vi "LS218_AIDE.vi"() -> ()   [LabVIEW 2014]
panel:
  in  "Bouton OK":bool
  # "VÉRIFICATION DU DÉBIT DU LAKESHORE 218:"
  # "Le débit doit être le même entre le LS218 et le logiciel d'acquisition"
  # "VÉRIFICATION DU CABLE SÉRIE:"
  # "La liaison série est RS232 mais le câble de liaison n'est pas standard, il doit être FEMELLE des deux côtés et doit respecter le brochage suivant :"
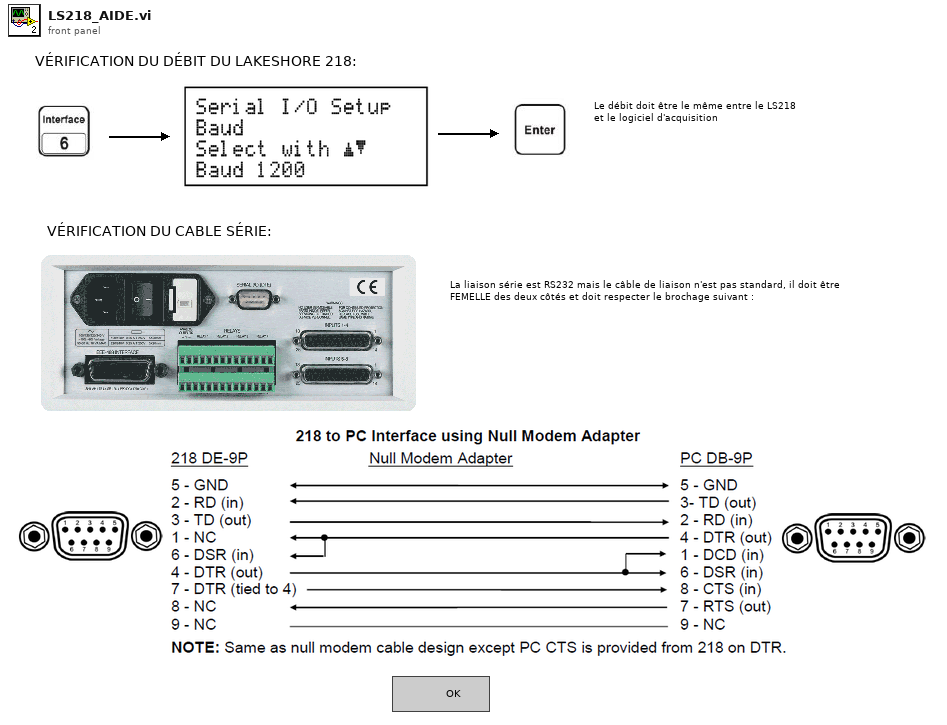
[diagram p1: front panel]
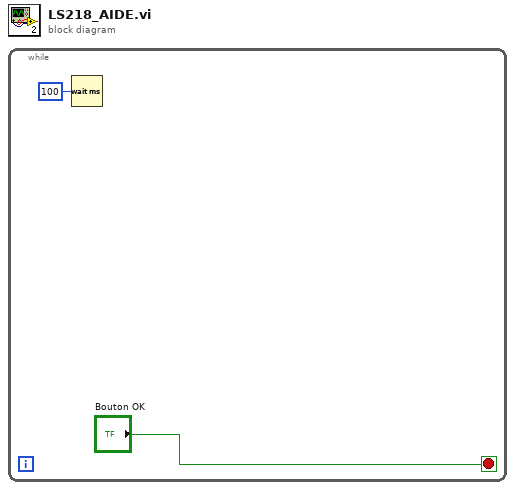
[diagram p0: block diagram]
diagram:
  n1 = while {
    stop <- "Bouton OK" stop-if-true
    n2 = Wait (ms)(milliseconds to wait=u32 100 ("attente (ms)")) -> ()  [unwired: 1 out]
  }
